vi "File.Parse CSV with Quotes.vi"() -> ()   [LabVIEW 2024]
panel:
  out "2D Data":string[][](array[string])
  in  "CSV Data":string
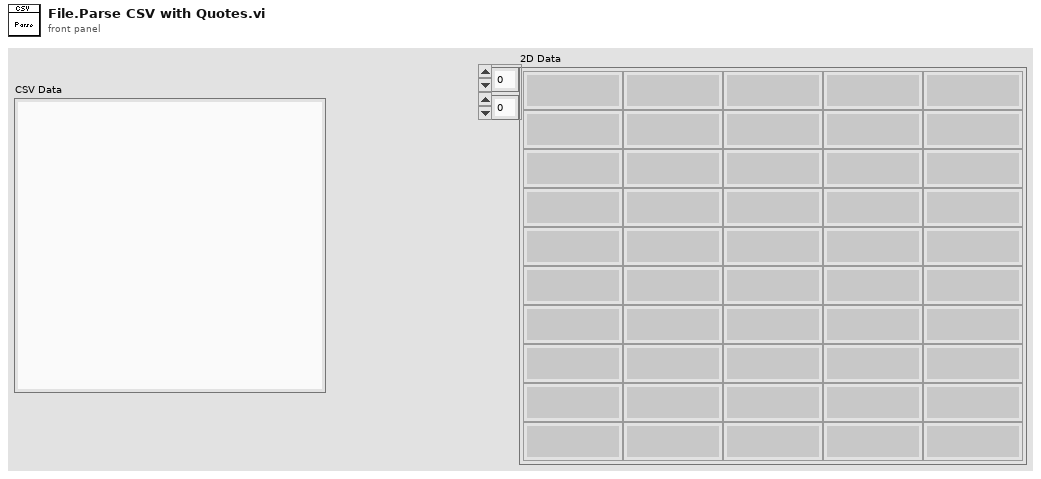
[diagram p1: front panel]
types:
  T1 = enum16{"New Element", "Look for Comma", "Look for End Quote"}
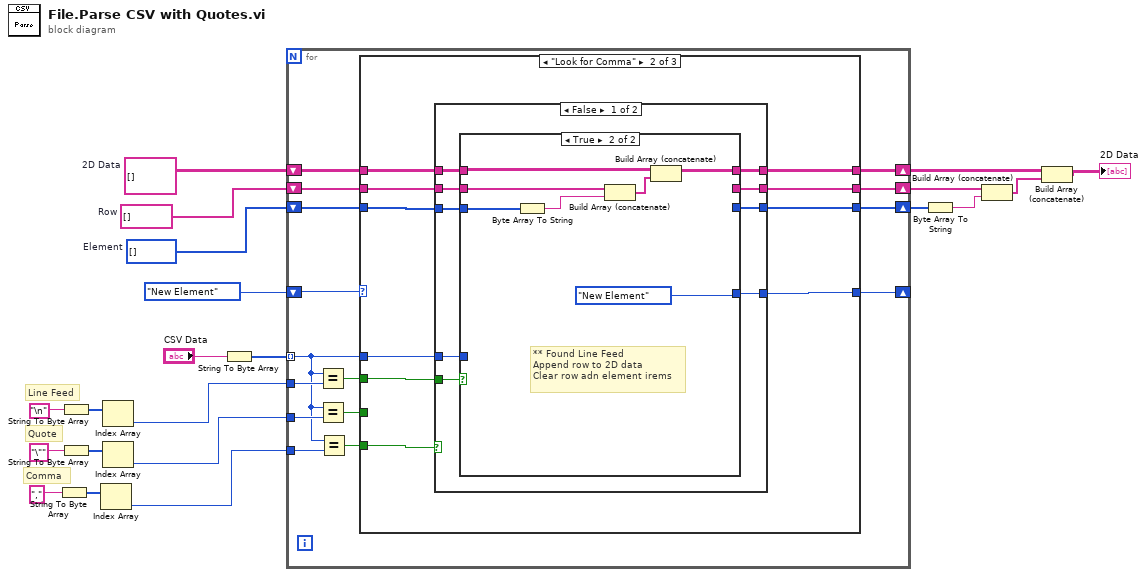
[diagram p0: block diagram]
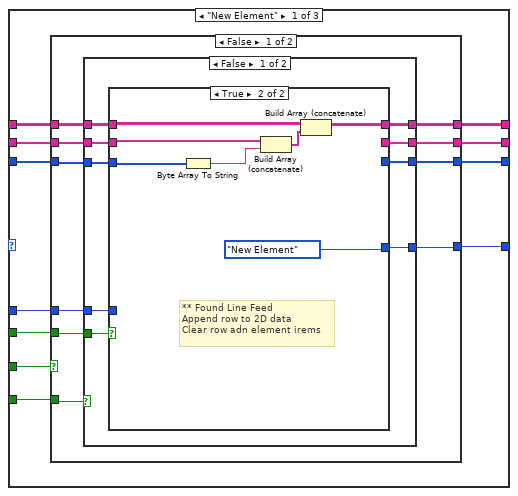
[diagram p2: hidden frame]
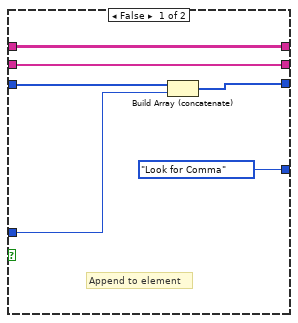
[diagram p3: hidden frame]
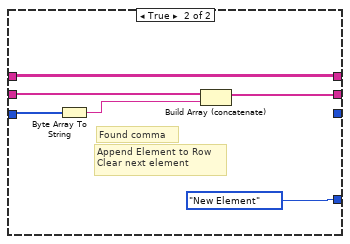
[diagram p4: hidden frame]
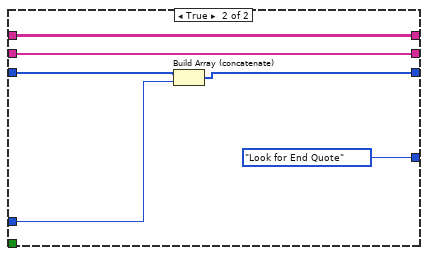
[diagram p5: hidden frame]
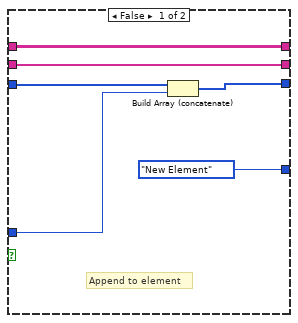
[diagram p6: hidden frame]
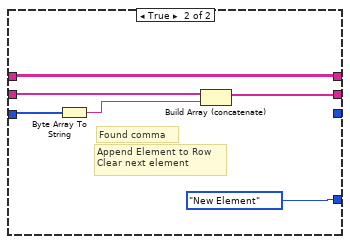
[diagram p7: hidden frame]
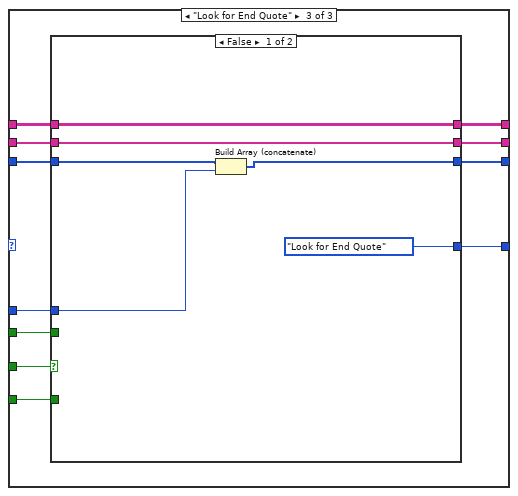
[diagram p8: hidden frame]
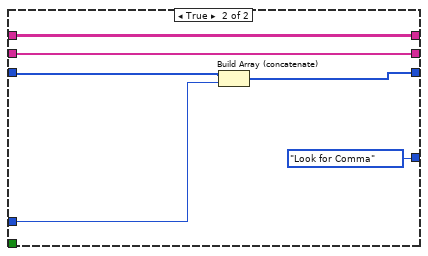
[diagram p9: hidden frame]
diagram:
  w8 = string[][] []  # 2D Data
  w7 = string[] []  # Row
  w19 = u8[] []  # Element
  # "Comma"
  # "Quote"
  # "Line Feed"
  n1 = String To Byte Array(string=",") -> (unsigned byte array=w13:u8[])
  n2 = String To Byte Array(string="\n") -> (unsigned byte array=w17:u8[])
  n3 = String To Byte Array(string="\"") -> (unsigned byte array=w16:u8[])
  n4 = Index Array(array=w13) -> (element=w10:u8)  [unwired: 1 in]
  n5 = Index Array(array=w17) -> (element=w12:u8)  [unwired: 1 in]
  n6 = Index Array(array=w16) -> (element=w11:u8)  [unwired: 1 in]
  n7 = String To Byte Array(string="CSV Data") -> (unsigned byte array=w20:u8[])
  n8 = for {
    shift-right: [w31] -> w2
    shift-left: w7 -> [w34]
    tunnel: w20 -> [w27] mode=indexing
    shift-right: [w30] -> w4
    shift-left: w19 -> [w33]
    shift-right: [w22] -> _
    shift-left: T1."New Element" -> [w36]
    tunnel: w12 -> [w29]
    tunnel: w11 -> [w28]
    tunnel: w10 -> [w26]
    shift-right: [w32] -> w6
    shift-left: w8 -> [w35]
    n9 = Equal?(x=w27, y=w29) -> (x = y?=w25:bool)
    n10 = Equal?(x=w27, y=w28) -> (x = y?=w24:bool)
    n11 = Equal?(x=w27, y=w26) -> (x = y?=w23:bool)
    n12 = case shown="\"Look for Comma\"" w36 {
      tunnel: w35 -> [w43 w98 w136]
      tunnel: w34 -> [w42 w97 w135]
      tunnel: w33 -> [w41 w96 w134]
      tunnel: [w40 w95 w133] -> w32
      tunnel: [w39 w94 w132] -> w31
      tunnel: [w38 w93 w131] -> w30
      tunnel: w27 -> [w37 w92 w130]
      tunnel: w25 -> [w45 w100 w138]
      tunnel: w24 -> [w47 _ w140]
      tunnel: w23 -> [w44 w99 w137]
      tunnel: [w46 w101 w139] -> w22
      frame "New Element" {
        n13 = case shown="False" w47 {
          tunnel: [w48 T1."Look for End Quote"] -> w46
          tunnel: w45 -> [w53 _]
          tunnel: w44 -> [w57 _]
          tunnel: w43 -> [w50 w91]
          tunnel: w42 -> [w52 w90]
          tunnel: w41 -> [w56 w87]
          tunnel: [w49 w91] -> w40
          tunnel: [w51 w90] -> w39
          tunnel: [w54 w86] -> w38
          tunnel: w37 -> [w55 w88]
          frame False {
            n14 = case shown="False" w57 {
              tunnel: w56 -> [w66 w81]
              tunnel: w55 -> [w65 _]
              tunnel: [w64 _] -> w54
              tunnel: w53 -> [w63 _]
              tunnel: w52 -> [w62 w82]
              tunnel: [w61 w83] -> w51
              tunnel: w50 -> [w60 w84]
              tunnel: [w59 w84] -> w49
              tunnel: [w58 T1."New Element"] -> w48
              frame False {
                n15 = case shown="True" w63 {
                  tunnel: w66 -> [w72 w74]
                  tunnel: w65 -> [w71 _]
                  tunnel: [w70 _] -> w64
                  tunnel: w62 -> [w69 w75]
                  tunnel: [w69 _] -> w61
                  tunnel: w60 -> [w68 w79]
                  tunnel: [w68 w78] -> w59
                  tunnel: [T1."Look for Comma" T1."New Element"] -> w58
                  frame False {
                    # "Append to element"
                    n16 = Build Array (concatenate)(w72, w71) -> (w70:u8[])
                  }
                  frame True {
                    # "** Found Line Feed\nAppend row to 2D data\nClear row adn element irems"
                    n17 = Byte Array To String(unsigned byte array=w74) -> (string=w73:string)
                    n18 = Build Array (concatenate)(w75, w73) -> (w76:string[])
                    n19 = Build Array (concatenate)(w79, w76) -> (w78:string[][])
                  }
                }
              }
              frame True {
                # "Found comma"
                # "Append Element to Row\nClear next element"
                n20 = Byte Array To String(unsigned byte array=w81) -> (string=w85:string)
                n21 = Build Array (concatenate)(w82, w85) -> (w83:string[])
              }
            }
          }
          frame True {
            n22 = Build Array (concatenate)(w87, w88) -> (w86:u8[])
          }
        }
      }
      frame "Look for Comma" {
        n23 = case shown="False" w99 {
          tunnel: w96 -> [w110 w125]
          tunnel: w92 -> [w109 _]
          tunnel: [w108 _] -> w93
          tunnel: w100 -> [w107 _]
          tunnel: w97 -> [w106 w126]
          tunnel: [w105 w127] -> w94
          tunnel: w98 -> [w104 w128]
          tunnel: [w103 w128] -> w95
          tunnel: [w102 T1."New Element"] -> w101
          frame False {
            n24 = case shown="True" w107 {
              tunnel: w110 -> [w116 w118]
              tunnel: w109 -> [w115 _]
              tunnel: [w114 _] -> w108
              tunnel: w106 -> [w113 w119]
              tunnel: [w113 _] -> w105
              tunnel: w104 -> [w112 w123]
              tunnel: [w112 w122] -> w103
              tunnel: [T1."New Element" T1."New Element"] -> w102
              frame False {
                # "Append to element"
                n25 = Build Array (concatenate)(w116, w115) -> (w114:u8[])
              }
              frame True {
                # "** Found Line Feed\nAppend row to 2D data\nClear row adn element irems"
                n26 = Byte Array To String(unsigned byte array=w118) -> (string=w117:string)
                n27 = Build Array (concatenate)(w119, w117) -> (w120:string[])
                n28 = Build Array (concatenate)(w123, w120) -> (w122:string[][])
              }
            }
          }
          frame True {
            # "Found comma"
            # "Append Element to Row\nClear next element"
            n29 = Byte Array To String(unsigned byte array=w125) -> (string=w129:string)
            n30 = Build Array (concatenate)(w126, w129) -> (w127:string[])
          }
        }
      }
      frame "Look for End Quote" {
        n31 = case shown="False" w140 {
          tunnel: [T1."Look for End Quote" T1."Look for Comma"] -> w139
          tunnel: w138 -> [_ _]
          tunnel: w137 -> [_ _]
          tunnel: w136 -> [w146 w152]
          tunnel: w135 -> [w145 w151]
          tunnel: w134 -> [w142 w150]
          tunnel: [w146 w152] -> w133
          tunnel: [w145 w151] -> w132
          tunnel: [w141 w148] -> w131
          tunnel: w130 -> [w143 w149]
          frame False {
            n32 = Build Array (concatenate)(w142, w143) -> (w141:u8[])
          }
          frame True {
            n33 = Build Array (concatenate)(w150, w149) -> (w148:u8[])
          }
        }
      }
    }
  }
  n34 = Byte Array To String(unsigned byte array=w4) -> (string=w3:string)
  n35 = Build Array (concatenate)(w2, w3) -> (w1:string[])
  n36 = Build Array (concatenate)(w6, w1) -> (→"2D Data":string[][])
